vi "SubVI.vi"(4 "Array Control In":bool[][](array[boolean]), 5 "Error In":errorcluster) -> (1 "Array Indicator Out":bool[][](array[boolean]), 2 "Error Out":errorcluster)   [LabVIEW 2018]
panel:
  in  "Close SubVI":bool
  # "To set the subVI to open its front panel when called:\n1. Go to File»VI Properties\n2. In the Category drop-down menu choose \"Window Appearance\" \n3. Click the \"Custom\" button\n4. Place checkmarks in the Show front panel when called and Close afterwards if originally closed checkboxes.\n\nThe predefined option \"Dialog\" also behaves this way"
  # "make sure both arrays have set the Index Display values at (0, 0)"
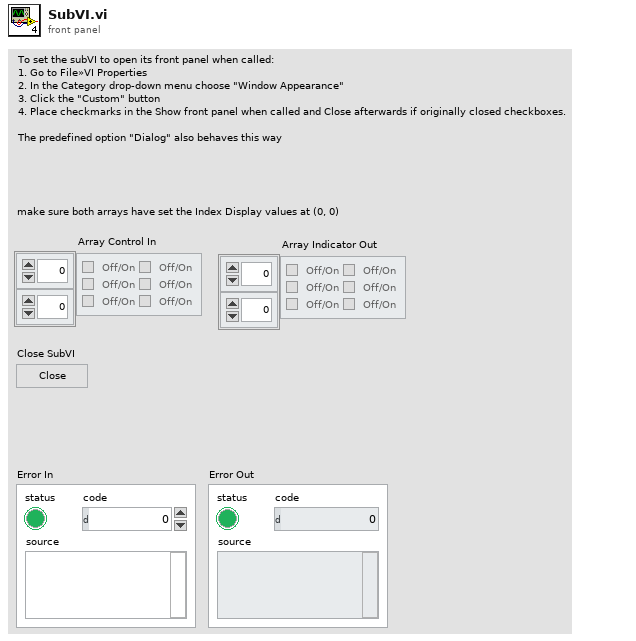
[diagram p1: front panel]
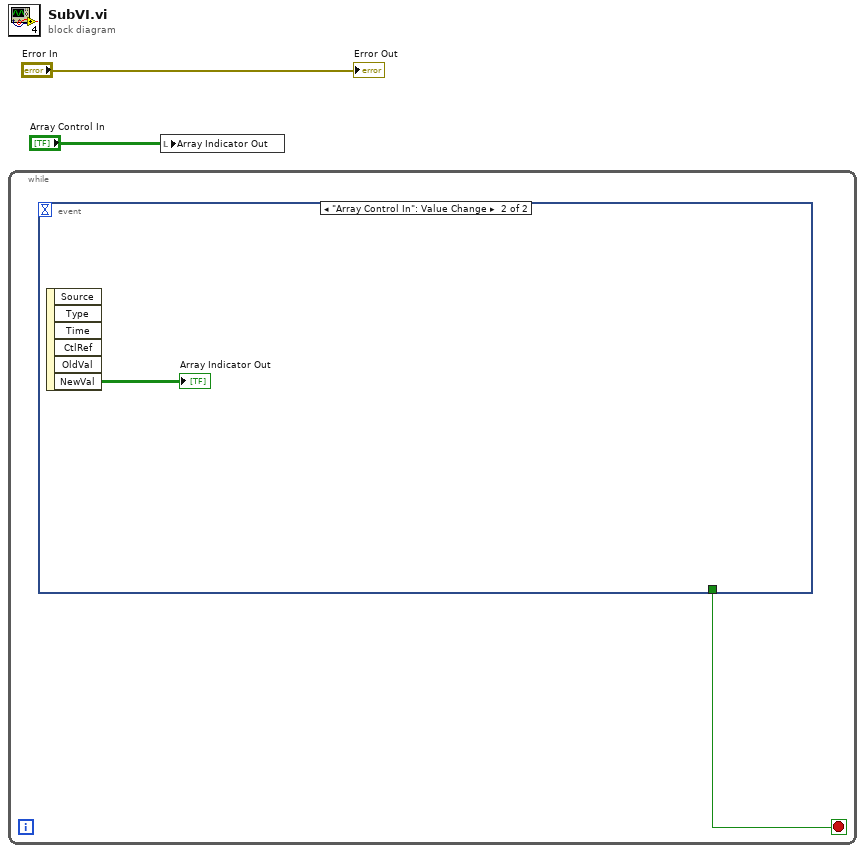
[diagram p0: block diagram]
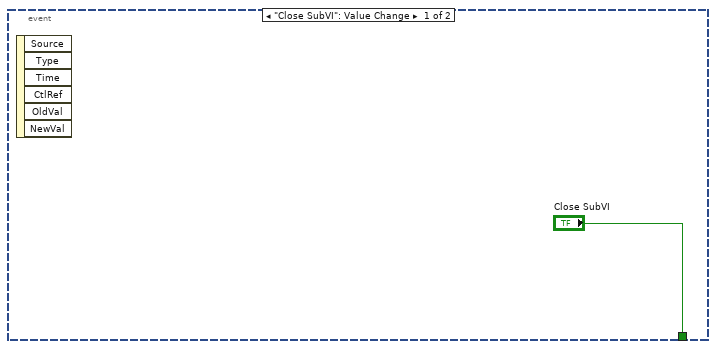
[diagram p2: hidden frame]
diagram:
  n1 = while {
    stop <- w3 stop-if-true
    n2 = event shown="[1] \"Array Control In\": Value Change" {
      selector: _ -> [_ _]
      dyn-events: _ -> [_ _]
      timeout: _ -> [_ _]
      tunnel: ["Close SubVI" _] -> w3
      event "Close SubVI": Value Change {
        n3 = event-data() -> ()  [unwired: 1 in, 6 out]
      }
      event "Array Control In": Value Change {
        n4 = event-data() -> ("NewVal"=→"Array Indicator Out":bool[][])  [unwired: 1 in, 5 out]
      }
    }
  }
  n5 = local write "Array Indicator Out"("Array Control In") -> ()
  "Error Out" <- "Error In"
